vi "HRR-SetID.vi"(8 "error in":errorcluster, 10 "ID":u8[](array[numeric]), 11 "FPGA VI Reference In":refnum<k20>) -> (0 "error out":errorcluster, 3 "FPGA VI Reference Out":refnum<k20>)   [LabVIEW 2019]
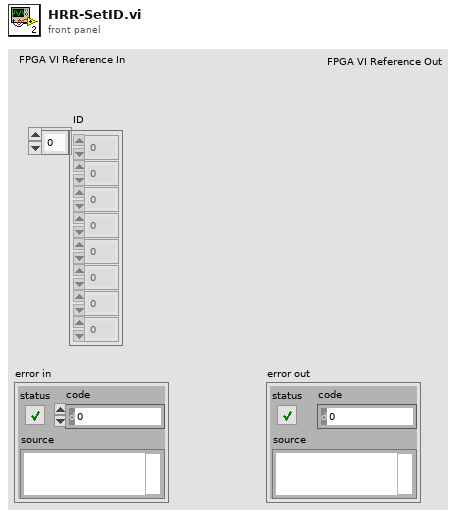
[diagram p1: front panel]
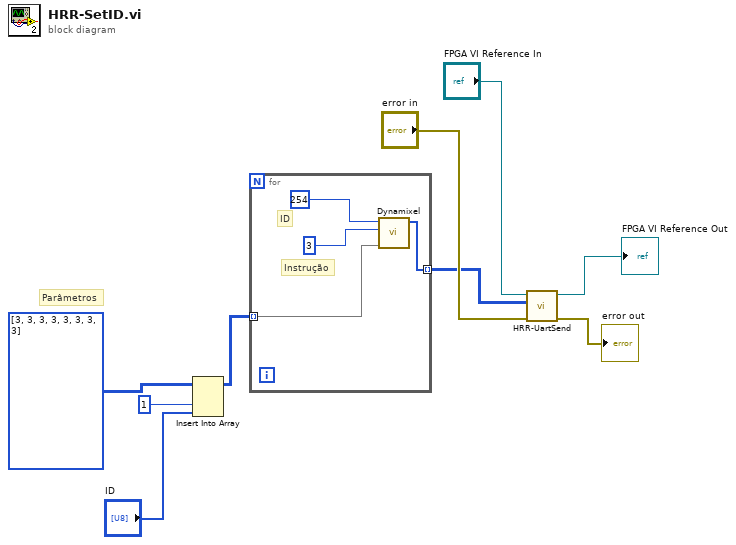
[diagram p0: block diagram]
diagram:
  # "Parâmetros"
  n1 = Insert Into Array(array=u8[][] [[3], [3], [3], [3], [3], [3], [3], [3]], index (col)=1 ("disabled index (col)"), new element="ID") -> (w5:u8[][])  [unwired: 1 in]
  n2 = for {
    tunnel: w5 -> [w11] mode=indexing
    tunnel: [w10] -> w2 mode=indexing
    # "Instrução"
    # "ID"
    n3 = call "Dynamixel.vi"("ID"=u8 254, "Instruction"=u8 3, "Array in"=w11) -> ("Array out"=w10:u8[])  [unwired: 7 in]
  }
  n4 = call "HRR-UartSend.vi"("error in (no error)"="error in", "Array"=w2, "Refnum in"="FPGA VI Reference In") -> ("error out"=→"error out":errorcluster, "Refnum out"=→"FPGA VI Reference Out":refnum<k20>)  [unwired: 7 in]
